vi "Periodic Tasks.vi"(8 "error in":errorcluster) -> ()   [LabVIEW 2019]
doc: "This VI runs in parallel to other tasks. It can contain as many user-defined periodic loops as you need. These can carry out PID or other sorts of timed response."
uses:
  Robot Global Data.vi
  <vilib>/Rock Robotics/WPI/Camera/WPI_CameraImageSize.ctl
  <vilib>/Rock Robotics/WPI/Camera/WPI_CameraFrameRate.ctl
  <vilib>/Rock Robotics/WPI/Camera/WPI_CameraWhite Balance Values.ctl
  <vilib>/Rock Robotics/WPI/Camera/WPI_CameraExposure Values.ctl
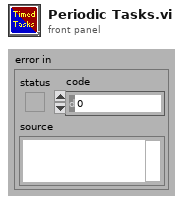
[diagram p1: front panel]
types:
  T1 = typedef "WPI_CameraExposure Values.ctl" = enum16{"Auto", "Flicker-free 50 Hz", "Flicker-free 60 Hz", "Hold current", "Custom"}
  T2 = typedef "WPI_CameraWhite Balance Values.ctl" = enum16{"Auto", "Fixed indoor", "Fixed outdoor 1", "Fixed outdoor 2", "Fixed fluorescent 1", "Fixed fluorescent 2", "Hold current", "Custom"}
  T3 = typedef "WPI_CameraFrameRate.ctl" = u32
  T4 = typedef "WPI_CameraImageSize.ctl" = enum16{"640x480", "320x240", "160x120", "Custom"}
  T5 = typedef "WPI_CameraDevRef.ctl" = cluster{"Camera Address":string, "CameraStatus":errorcluster}
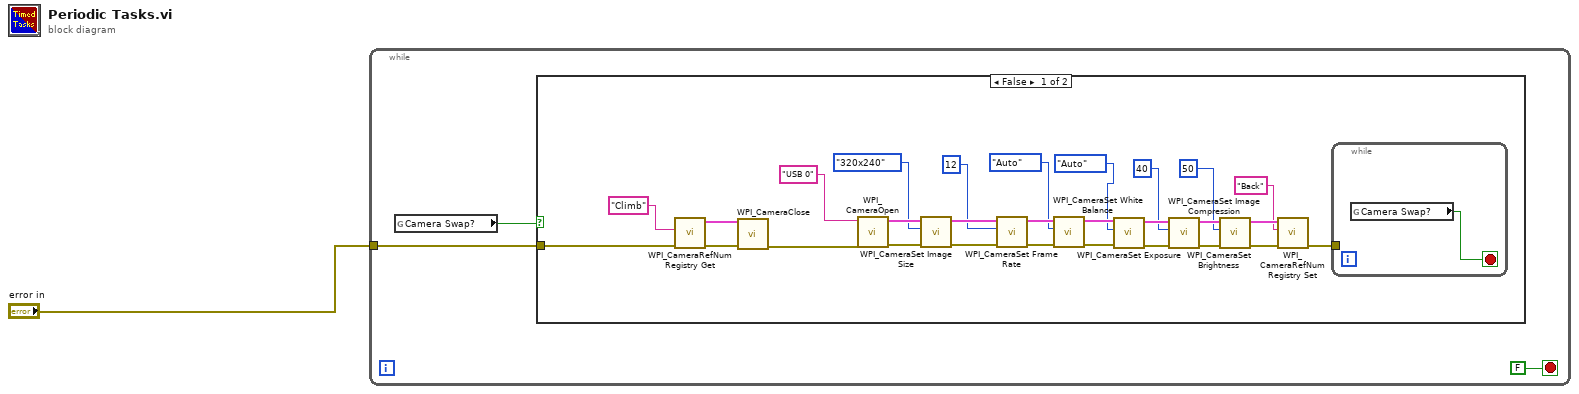
[diagram p0: block diagram]
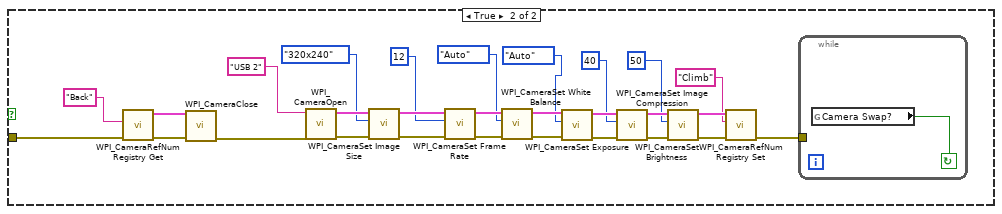
[diagram p2: hidden frame]
diagram:
  n1 = while {
    tunnel: "error in" -> [w2]
    stop <- FALSE stop-if-true
    n2 = global read "Robot Global Data.vi" "Camera Swap?"() -> (w4:bool)
    n3 = case shown="False" w4 {
      tunnel: w2 -> [w6 w59]
      frame False {
        n4 = call <vilib>:"WPI_CameraRefNum Registry Get.vi"("error in (no error)"=w6, "refnum name"="Climb") -> ("error out"=w17:errorcluster, "CameraDevRef"=w16:T5)  [unwired: 8 in]
        n5 = call <vilib>:"WPI_CameraClose.vi"("error in (no error)"=w17, "CameraDevRef"=w16) -> ("error out"=w32:errorcluster)  [unwired: 9 in]
        n6 = call <vilib>:"WPI_CameraOpen.vi"("error in (no error)"=w32, "Camera Address"="USB 0") -> ("error out"=w18:errorcluster, "CameraDevRef"=w19:T5)  [unwired: 8 in]
        n7 = call <vilib>:"WPI_CameraSet Image Size.vi"("error in (no error)"=w18, "Image Size"=WPI_CameraImageSize."320x240", "CameraDevRef"=w19) -> ("error out"=w20:errorcluster, "CameraDevRef Out"=w21:T5)  [unwired: 7 in]
        n8 = call <vilib>:"WPI_CameraSet Frame Rate.vi"("error in (no error)"=w20, "Frame Rate (fps)"=T3 12, "CameraDevRef"=w21) -> ("error out"=w22:errorcluster, "CameraDevRef Out"=w23:T5)  [unwired: 7 in]
        n9 = call <vilib>:"WPI_CameraSet White Balance.vi"("error in (no error)"=w22, "White Balance"=WPI_CameraWhite_Balance_Values."Auto", "CameraDevRef"=w23) -> ("error out"=w24:errorcluster, "CameraDevRef Out"=w25:T5)  [unwired: 7 in]
        n10 = call <vilib>:"WPI_CameraSet Exposure.vi"("error in (no error)"=w24, "Exposure"=WPI_CameraExposure_Values."Auto", "CameraDevRef"=w25) -> ("error out"=w26:errorcluster, "CameraDevRef Out"=w27:T5)  [unwired: 7 in]
        n11 = call <vilib>:"WPI_CameraSet Image Compression.vi"("error in (no error)"=w26, "Compression"=40, "CameraDevRef"=w27) -> ("error out"=w28:errorcluster, "CameraDevRef Out"=w29:T5)  [unwired: 7 in]
        n12 = call <vilib>:"WPI_CameraSet Brightness.vi"("error in (no error)"=w28, "Brightness"=50, "CameraDevRef"=w29) -> ("error out"=w30:errorcluster, "CameraDevRef Out"=w31:T5)  [unwired: 7 in]
        n13 = call <vilib>:"WPI_CameraRefNum Registry Set.vi"("error in (no error)"=w30, "refnum name"="Back", "CameraDevRef"=w31) -> ("error out"=w5:errorcluster)  [unwired: 7 in, 1 out]
        n14 = while {
          tunnel: w5 -> [_]
          stop <- w33 stop-if-true
          n15 = global read "Robot Global Data.vi" "Camera Swap?"() -> (w33:bool)
        }
      }
      frame True {
        n16 = call <vilib>:"WPI_CameraRefNum Registry Get.vi"("error in (no error)"=w59, "refnum name"="Back") -> ("error out"=w60:errorcluster, "CameraDevRef"=w61:T5)  [unwired: 8 in]
        n17 = call <vilib>:"WPI_CameraClose.vi"("error in (no error)"=w60, "CameraDevRef"=w61) -> ("error out"=w35:errorcluster)  [unwired: 9 in]
        n18 = call <vilib>:"WPI_CameraOpen.vi"("error in (no error)"=w35, "Camera Address"="USB 2") -> ("error out"=w57:errorcluster, "CameraDevRef"=w56:T5)  [unwired: 8 in]
        n19 = call <vilib>:"WPI_CameraSet Image Size.vi"("error in (no error)"=w57, "Image Size"=WPI_CameraImageSize."320x240", "CameraDevRef"=w56) -> ("error out"=w55:errorcluster, "CameraDevRef Out"=w54:T5)  [unwired: 7 in]
        n20 = call <vilib>:"WPI_CameraSet Frame Rate.vi"("error in (no error)"=w55, "Frame Rate (fps)"=T3 12, "CameraDevRef"=w54) -> ("error out"=w53:errorcluster, "CameraDevRef Out"=w52:T5)  [unwired: 7 in]
        n21 = call <vilib>:"WPI_CameraSet White Balance.vi"("error in (no error)"=w53, "White Balance"=WPI_CameraWhite_Balance_Values."Auto", "CameraDevRef"=w52) -> ("error out"=w51:errorcluster, "CameraDevRef Out"=w50:T5)  [unwired: 7 in]
        n22 = call <vilib>:"WPI_CameraSet Exposure.vi"("error in (no error)"=w51, "Exposure"=WPI_CameraExposure_Values."Auto", "CameraDevRef"=w50) -> ("error out"=w49:errorcluster, "CameraDevRef Out"=w48:T5)  [unwired: 7 in]
        n23 = call <vilib>:"WPI_CameraSet Image Compression.vi"("error in (no error)"=w49, "Compression"=40, "CameraDevRef"=w48) -> ("error out"=w47:errorcluster, "CameraDevRef Out"=w46:T5)  [unwired: 7 in]
        n24 = call <vilib>:"WPI_CameraSet Brightness.vi"("error in (no error)"=w47, "Brightness"=50, "CameraDevRef"=w46) -> ("error out"=w38:errorcluster, "CameraDevRef Out"=w37:T5)  [unwired: 7 in]
        n25 = call <vilib>:"WPI_CameraRefNum Registry Set.vi"("error in (no error)"=w38, "refnum name"="Climb", "CameraDevRef"=w37) -> ("error out"=w34:errorcluster)  [unwired: 7 in, 1 out]
        n26 = while {
          tunnel: w34 -> [_]
          stop <- w62 continue-if-true
          n27 = global read "Robot Global Data.vi" "Camera Swap?"() -> (w62:bool)
        }
      }
    }
  }
